vi "Set Loop Type.vi"(8 "error in (no error)":errorcluster, 9 "Loop Type":string, 11 "Port In":T1) -> (0 "error out":errorcluster, 3 "Port Out":T1)   [LabVIEW 2021]
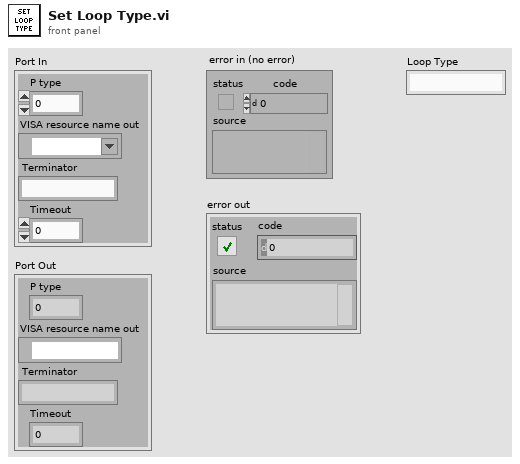
[diagram p1: front panel]
types:
  T1 = cluster{"P type":u16, "VISA resource name out":refnum<visa-resource-name>, " Terminator":string, "Timeout":i32}
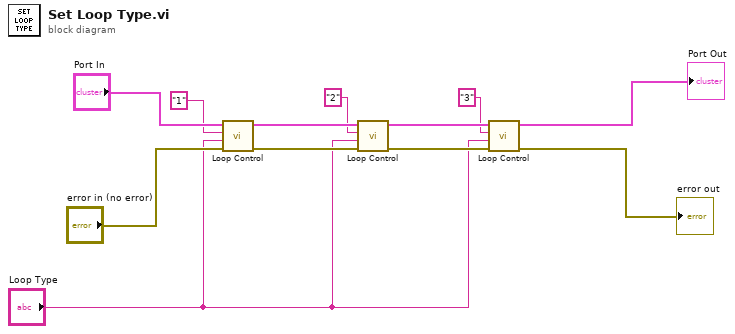
[diagram p0: block diagram]
diagram:
  n1 = call "Loop Control.vi"("error in (no error)"="error in (no error)", "Loop Type"="Loop Type", "Controller #"="1", "Port In"="Port In") -> ("error out"=w9:errorcluster, "Port Out"=w6:T1)  [unwired: 6 in]
  n2 = call "Loop Control.vi"("error in (no error)"=w9, "Loop Type"="Loop Type", "Controller #"="2", "Port In"=w6) -> ("error out"=w8:errorcluster, "Port Out"=w5:T1)  [unwired: 6 in]
  n3 = call "Loop Control.vi"("error in (no error)"=w8, "Loop Type"="Loop Type", "Controller #"="3", "Port In"=w5) -> ("error out"=→"error out":errorcluster, "Port Out"=→"Port Out":T1)  [unwired: 6 in]
